vi "Rotate_X_degrees(SubVI).vi"(1 "Encoder Delay (msec)":u32, 7 "Motor (Port A)":T1 items=["Port A", "Port B", "Port C", "Port D"], 8 "Power/Speed 1":i8, 9 "Position Change (180)":i32, 11 "BrickReference in":T2) -> (3 "BrickReference out":T2)   [LabVIEW 2014]
uses:
  <vilib>/NXT/Subs/LVHSConnector.ctl
  <vilib>/NXT/LegoClasses/BrickReference/BrickReference.lvclass
  <vilib>/NXT/Block Support/NXT_OutputPort.ctl
  <vilib>/NXT/NXTIO Xnodes/NXTIONodeSubVIs/NXTStopMotors.vi
  <vilib>/NXT/Dual Mode Library/Waits/Wait_Num(msec).vi
  <vilib>/NXT/NXTIO Xnodes/NXTIONodeSubVIs/LEGOResetMotors.vi
  <vilib>/NXT/NXTIO Xnodes/NXTIONodeSubVIs/NXTMoveMotors.vi
  <vilib>/NXT/Dual Mode Library/Waits/Wait_Rotation.vi
  <vilib>/NXT/NXTIO Xnodes/NXTIOXNode/NXTIO.xnode
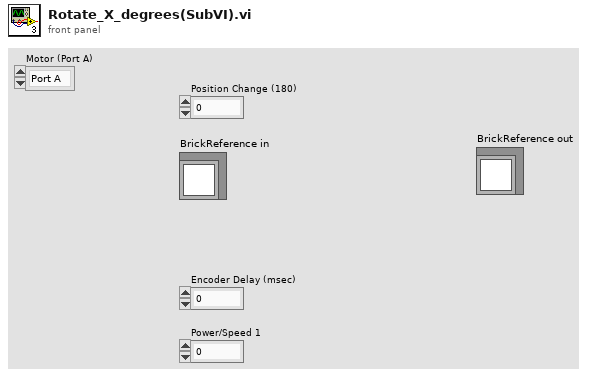
[diagram p1: front panel]
types:
  T1 = typedef "NXT_OutputPort.ctl" = u8
  T2 = typedef "LVHSConnector.ctl" = refnum<class "BrickReference.lvclass">
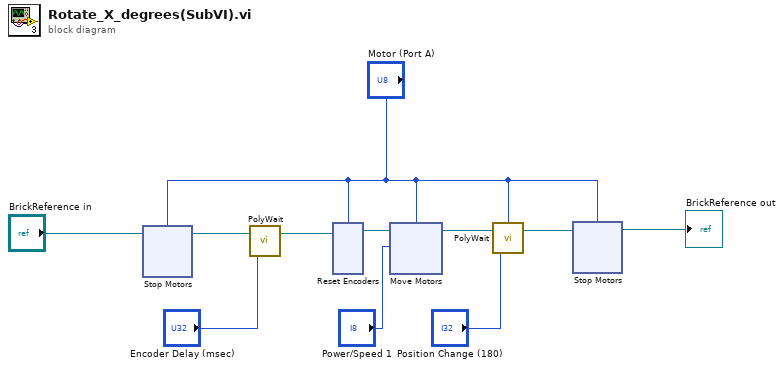
[diagram p0: block diagram]
diagram:
  n1 = xnode "Stop Motors"("Motors"="Motor (Port A)", "NXT/EV3"="BrickReference in") -> ("NXT/EV3"=w2:T2)
  n2 = call-poly <vilib>:"PolyWait.vi"("Time (100 msec)"="Encoder Delay (msec)", "NXT/EV3"=w2) -> ("NXT/EV3"=w3:T2)  [unwired: 2 in]
  n3 = xnode "Reset Encoders"("Motors"="Motor (Port A)", "NXT/EV3"=w3) -> ("NXT/EV3"=w4:T2)
  n4 = xnode "Move Motors"("Power/Speed 1"="Power/Speed 1", "Motors"="Motor (Port A)", "NXT/EV3"=w4) -> ("NXT/EV3"=w5:T2)
  n5 = call-poly <vilib>:"PolyWait.vi"("Position Change (180)"="Position Change (180)", "NXT/EV3"=w5, "Port (Port A)"="Motor (Port A)") -> ("NXT/EV3"=w6:T2)  [unwired: 1 in]
  n6 = xnode "Stop Motors"("Motors"="Motor (Port A)", "NXT/EV3"=w6) -> ("NXT/EV3"=→"BrickReference out":T2)
